vi "SPARK Get Soft Limit Status.vi"   [LabVIEW 2023]
doc: "Get the status of a soft limit on the SPARK."
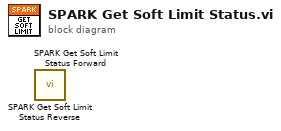
[diagram p0: block diagram]
diagram:
  n1 = call "SPARK Get Soft Limit Status Reverse.vi"() -> ()  [unwired: 8 in, 4 out]
  n2 = call "SPARK Get Soft Limit Status Forward.vi"() -> ()  [unwired: 8 in, 4 out]
